vi "Main.vi"(11 "ROS_Master in":refnum<class "ROS_Master.lvclass">) -> ()   [LabVIEW 2013, in "ROS_Master.lvclass"]
uses:
  <userlib>/ROSforLV/ROS/Code/SubVIs/ROS_Master/ROS_Master.lvclass
  <userlib>/ROSforLV/ROS/Code/SubVIs/ROS_Master/ROS_Master.lvclass/ROS_Master.ctl
  <userlib>/ROSforLV/ROS/Code/_ROSDefinition.vi
panel:
  in  "stop":bool
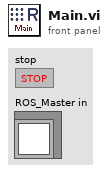
[diagram p1: front panel]
types:
  T1 = cluster{"Caller ID":string, "IP":string, "Msg Type":string, "Direction":enum16{"Publisher", "Subscriber"}, "Topic":string}
  T2 = cluster{"value":string, "value":string, "value":string}
  T3 = cluster{"Service":string, "Service IP":string, "Caller IP":string, "Caller ID":string}[]
  T4 = cluster{"Service":string, "Service IP":string, "Caller IP":string, "Caller ID":string}
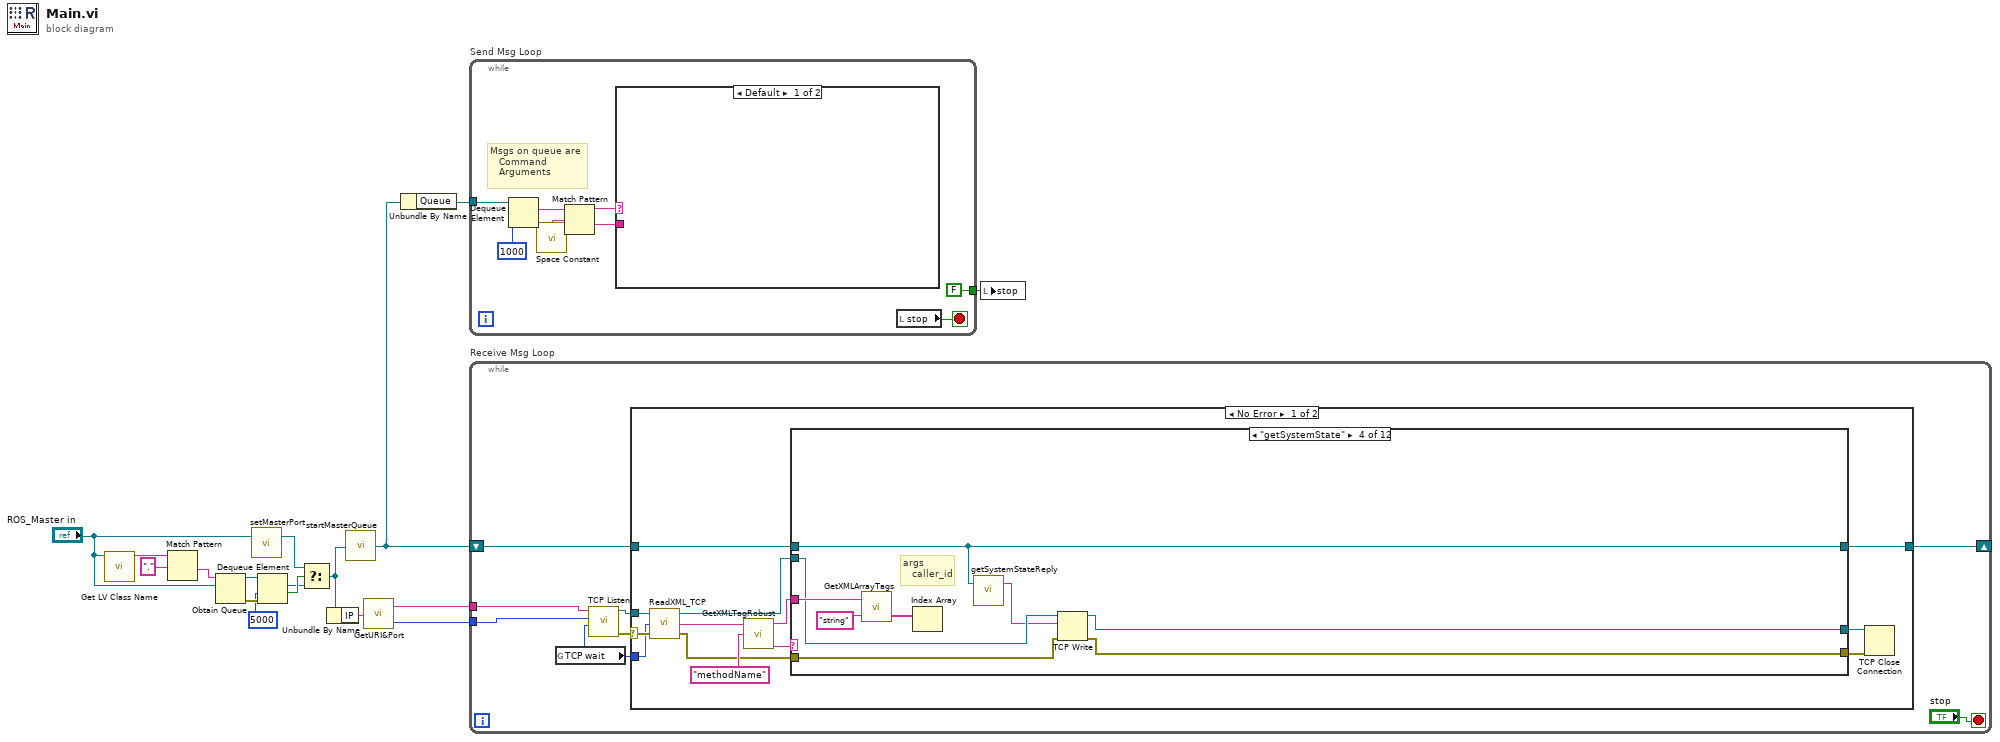
[diagram p0: block diagram]
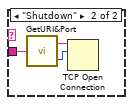
[diagram p2: hidden frame]
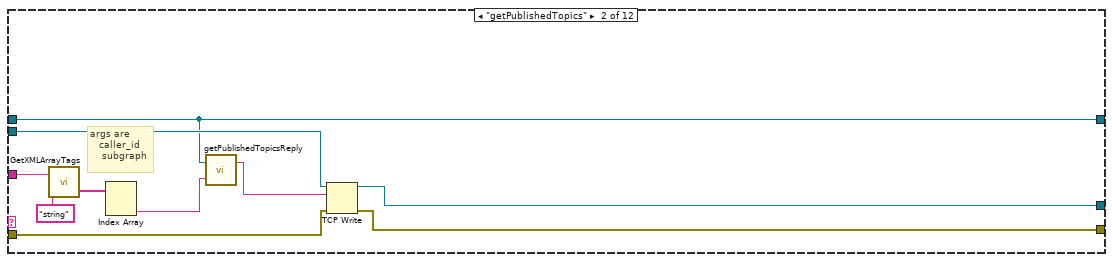
[diagram p4: hidden frame]
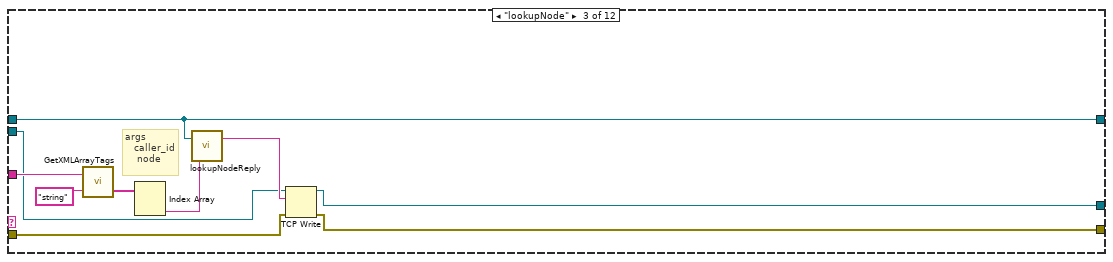
[diagram p5: hidden frame]
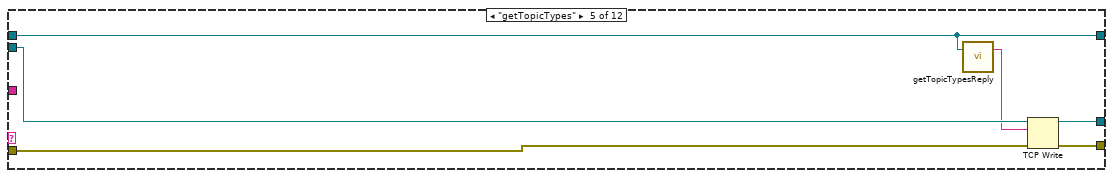
[diagram p6: hidden frame]
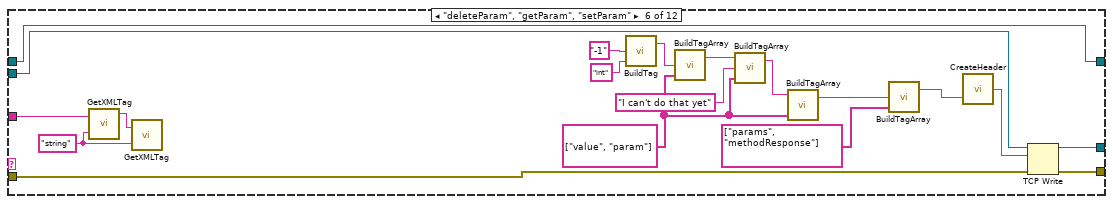
[diagram p7: hidden frame]
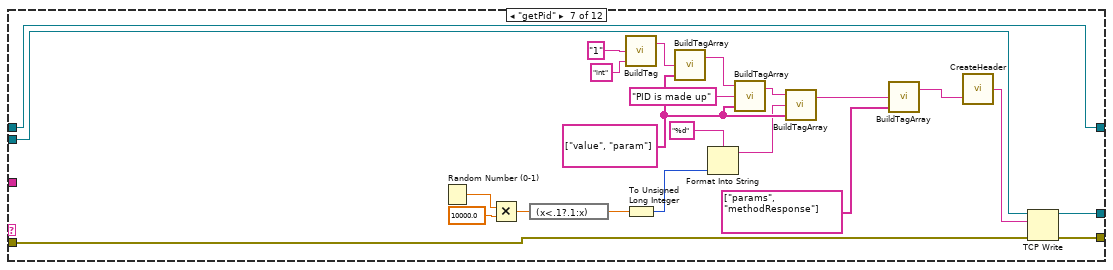
[diagram p8: hidden frame]
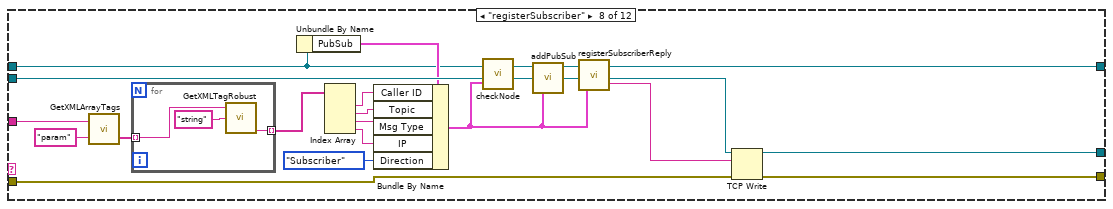
[diagram p9: hidden frame]
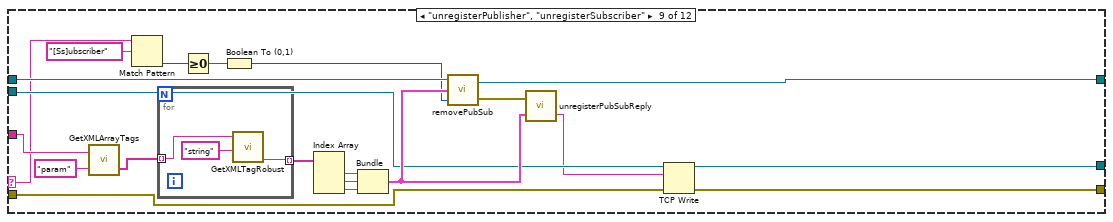
[diagram p10: hidden frame]
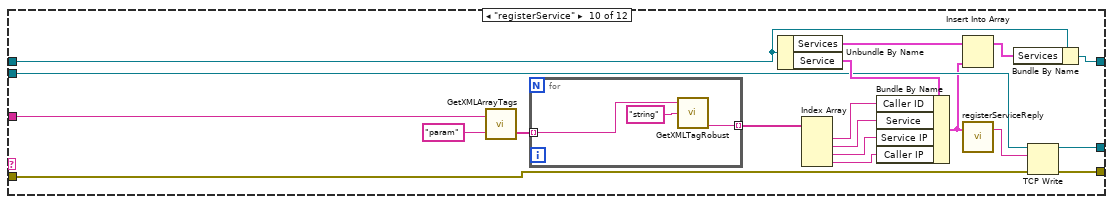
[diagram p11: hidden frame]
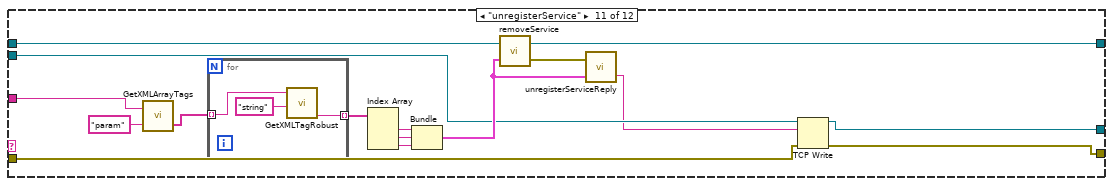
[diagram p12: hidden frame]
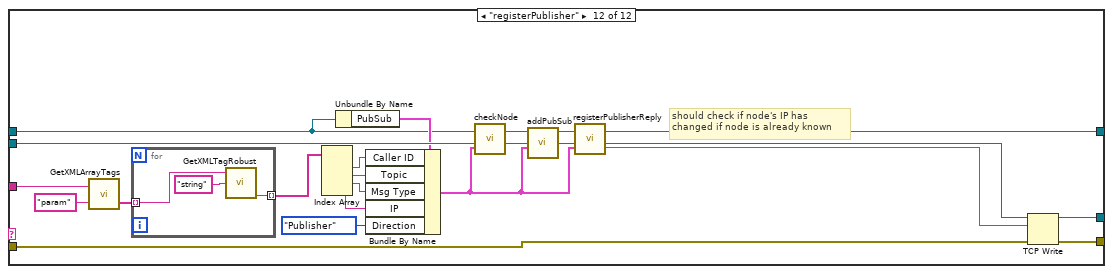
[diagram p13: hidden frame]
diagram:
  n1 = call <vilib>:"Get LV Class Name.vi"("object"="ROS_Master in") -> ("class name"=w14:string)  [unwired: 9 in, 1 out]
  n2 = Match Pattern(string=w14, regular expression=".") -> (after substring=w12:string)  [unwired: 1 in, 3 out]
  n3 = Obtain Queue(name (unnamed)=w12, element data type="ROS_Master in") -> (queue out=w10:refnum<queue>, error out=w11:errorcluster)  [unwired: 3 in, 1 out]
  n4 = call <userlib>:"setMasterPort.vi"("ROS_Master.lvclass in"="ROS_Master in") -> ("ROS_Master.lvclass out"=w6:refnum<class "ROS_Master.lvclass">)  [unwired: 2 in]
  n5 = Dequeue Element(queue=w10, timeout in ms (-1)=5000, error in (no error)=w11) -> (element=w5:refnum<class "ROS_Master.lvclass">, timed out?=w9:bool)  [unwired: 2 out]
  n6 = Select(t=w6, s=w9, f=w5) -> (s? t:f=w4:refnum<class "ROS_Master.lvclass">)
  n7 = Unbundle By Name(w4) -> ("IP"=w17:string)
  n8 = call <userlib>:"startMasterQueue.vi"("ROS_Master in"=w4) -> ("ROS_Master out"=w2:refnum<class "ROS_Master.lvclass">)
  n9 = call <userlib>:"GetURI&Port.vi"("URI in"=w17) -> ("Port"=w15:u16, "URI"=w16:string)
  n10 = Unbundle By Name(w2) -> ("Queue"=w1:refnum<queue>)
  n11 = while "Send Msg Loop" {
    tunnel: [FALSE ("stop")] -> w3
    tunnel: w1 -> [w23]
    stop <- w25 stop-if-true
    # "Msgs on queue are\n   Command\n   Arguments"
    n12 = Dequeue Element(queue=w23, timeout in ms (-1)=1000) -> (element=w21:string)  [unwired: 1 in, 3 out]
    n13 = call <vilib>:"Space Constant.vi"() -> ("String"=w20:string)
    n14 = Match Pattern(string=w21, regular expression=w20) -> (before substring=w19:string, after substring=w18:string)  [unwired: 1 in, 2 out]
    n15 = case shown="Default" w19 {
      tunnel: w18 -> [_ w28]
      frame Default {
      }
      frame "Shutdown" {
        n16 = call <userlib>:"GetURI&Port.vi"("URI in"=w28) -> ("Port"=w26:u16, "URI"=w27:string)
        n17 = TCP Open Connection(address=w27, remote port or service name=w26) -> ()  [unwired: 3 in, 2 out]
      }
    }
    n18 = local read "stop"() -> (w25:bool)
  }
  n19 = while "Receive Msg Loop" {
    shift-right: [w30] -> _
    shift-left: w2 -> [w31]
    tunnel: w16 -> [w34]
    tunnel: w15 -> [w33]
    stop <- "stop" stop-if-true
    n20 = global read "_ROSDefinition.vi" "TCP wait"() -> (w29:i32)
    n21 = call <vilib>:"TCP Listen.vi"("timeout ms (wait forever: -1)"=w29, "port"=w33, "service name"=w34) -> ("error out"=w35:errorcluster, "connection ID"=w32:refnum<k5>)  [unwired: 4 in, 3 out]
    n22 = case shown="No Error" w35 {
      selector: w35 -> [w48 _]
      tunnel: w32 -> [w49 _]
      tunnel: w31 -> [w43 w239]
      tunnel: [w42 w239] -> w30
      tunnel: w29 -> [w41 _]
      frame No Error {
        n23 = call <userlib>:"ReadXML_TCP.vi"("error in"=w48, "timeout ms (3000)"=w41, "connection ID in"=w49) -> ("error out"=w37:errorcluster, "data out"=w47:string, "connection ID out"=w40:refnum<k5>)
        n24 = call <userlib>:"GetXMLTagRobust.vi"("Tag"="methodName", "String"=w47) -> ("value"=w45:string, "String w/o Tag"=w44:string)  [unwired: 1 in, 2 out]
        n25 = case shown="\"getSystemState\"" w45 {
          selector: w45 -> [_ _ _ _ _ _ _ _ w156 _ _ _]
          tunnel: w44 -> [_ w62 w72 w81 _ w105 _ w148 w172 w194 w209 w235]
          tunnel: w43 -> [w52 w53 w63 w74 w82 w106 w129 w131 w165 w190 w206 w219]
          tunnel: [w52 w53 w63 w74 w82 w106 w129 w139 w164 w184 w198 w226] -> w42
          tunnel: w40 -> [w51 w58 w67 w78 w85 w92 w116 w144 w160 w181 w203 w231]
          tunnel: [w51 w55 w64 w75 w87 w90 w115 w143 w158 w179 w200 w229] -> w39
          tunnel: [w50 w54 w65 w76 w86 w89 w114 w141 w157 w178 w199 w228] -> w38
          tunnel: w37 -> [w50 w56 w66 w77 w84 w91 w113 w142 w161 w180 w202 w230]
          frame Default {
          }
          frame "getPublishedTopics" {
            # "args are\n   caller_id\n    subgraph"
            n26 = call <userlib>:"GetXMLArrayTags.vi"("ArrayTag"="string", "String"=w62) -> ("Array"=w60:string[])  [unwired: 1 out]
            n27 = Index Array(array=w60) -> (element #2=w59:string)  [unwired: 2 in, 1 out]
            n28 = call <userlib>:"getPublishedTopicsReply.vi"("Subgraph"=w59, "ROS_Master"=w53) -> ("XML"=w57:string)  [unwired: 1 in]
            n29 = TCP Write(connection ID=w58, data in=w57, error in (no error)=w56) -> (connection ID out=w55:refnum<k5>, error out=w54:errorcluster)  [unwired: 1 in, 1 out]
          }
          frame "lookupNode" {
            # "args\n   caller_id\n    node"
            n30 = call <userlib>:"GetXMLArrayTags.vi"("ArrayTag"="string", "String"=w72) -> ("Array"=w70:string[])  [unwired: 1 out]
            n31 = Index Array(array=w70) -> (element #2=w69:string)  [unwired: 2 in, 1 out]
            n32 = call <userlib>:"lookupNodeReply.vi"("node"=w69, "Master"=w63) -> ("XML"=w68:string)  [unwired: 1 in]
            n33 = TCP Write(connection ID=w67, data in=w68, error in (no error)=w66) -> (connection ID out=w64:refnum<k5>, error out=w65:errorcluster)  [unwired: 1 in, 1 out]
          }
          frame "getSystemState" {
            # "args\n   caller_id"
            n34 = call <userlib>:"GetXMLArrayTags.vi"("ArrayTag"="string", "String"=w81) -> ("Array"=w79:string[])  [unwired: 1 out]
            n35 = Index Array(array=w79) -> ()  [unwired: 1 in, 1 out]
            n36 = call <userlib>:"getSystemStateReply.vi"("ROS_Master in"=w74) -> ("XML"=w73:string)  [unwired: 2 in]
            n37 = TCP Write(connection ID=w78, data in=w73, error in (no error)=w77) -> (connection ID out=w75:refnum<k5>, error out=w76:errorcluster)  [unwired: 1 in, 1 out]
          }
          frame "getTopicTypes" {
            n38 = call <userlib>:"getTopicTypesReply.vi"("ROS_Master.lvclass in"=w82) -> ("Topics XML"=w83:string)  [unwired: 2 in]
            n39 = TCP Write(connection ID=w85, data in=w83, error in (no error)=w84) -> (connection ID out=w87:refnum<k5>, error out=w86:errorcluster)  [unwired: 1 in, 1 out]
          }
          frame "deleteParam", "getParam", "setParam" {
            w102 = string[] ["value", "param"] ("tags")
            w103 = "string" ("Tag")
            n40 = call <userlib>:"GetXMLTag.vi"("Tag"=w103, "String"=w105) -> ("String w/o Tag"=w104:string)  [unwired: 2 out]
            n41 = call <userlib>:"GetXMLTag.vi"("Tag"=w103, "String"=w104) -> ()  [unwired: 3 out]
            n42 = call <userlib>:"BuildTag.vi"("tag"="int", "value"="-1") -> ("string out"=w96:string)  [unwired: 2 in]
            n43 = call <userlib>:"BuildTagArray.vi"("tags"=w102, "value"=w96) -> ("string out"=w101:string)  [unwired: 2 in]
            n44 = call <userlib>:"BuildTagArray.vi"("tags"=w102, "value"="I can't do that yet", "string in"=w101) -> ("string out"=w100:string)  [unwired: 1 in]
            n45 = call <userlib>:"BuildTagArray.vi"("tags"=w102, "string in"=w100) -> ("string out"=w94:string)  [unwired: 2 in]
            n46 = call <userlib>:"BuildTagArray.vi"("tags"=string[] ["params", "methodResponse"], "value"=w94) -> ("string out"=w93:string)  [unwired: 2 in]
            n47 = call <userlib>:"CreateHeader.vi"("Content"=w93) -> ("XML"=w88:string)  [unwired: 1 in]
            n48 = TCP Write(connection ID=w92, data in=w88, error in (no error)=w91) -> (connection ID out=w90:refnum<k5>, error out=w89:errorcluster)  [unwired: 1 in, 1 out]
          }
          frame "getPid" {
            w128 = string[] ["value", "param"] ("tags")
            n49 = Random Number (0-1)() -> (number: 0 to 1=w125:dbl)
            n50 = Multiply(x=w125, y=10000.0) -> (x*y=w112:dbl)
            n51 = expression code="(x<.1?.1:x)"(w112) -> (w111:dbl)
            n52 = call <userlib>:"BuildTag.vi"("tag"="int", "value"="1") -> ("string out"=w107:string)  [unwired: 2 in]
            n53 = To Unsigned Long Integer(number=w111) -> (unsigned 32bit integer=w123:u32)
            n54 = call <userlib>:"BuildTagArray.vi"("tags"=w128, "value"=w107) -> ("string out"=w127:string)  [unwired: 2 in]
            n55 = Format Into String(format string="%d", w123) -> (resulting string=w121:string)  [unwired: 2 in, 1 out]
            n56 = call <userlib>:"BuildTagArray.vi"("tags"=w128, "value"="PID is made up", "string in"=w127) -> ("string out"=w126:string)  [unwired: 1 in]
            n57 = call <userlib>:"BuildTagArray.vi"("tags"=w128, "value"=w121, "string in"=w126) -> ("string out"=w120:string)  [unwired: 1 in]
            n58 = call <userlib>:"BuildTagArray.vi"("tags"=string[] ["params", "methodResponse"], "value"=w120) -> ("string out"=w118:string)  [unwired: 2 in]
            n59 = call <userlib>:"CreateHeader.vi"("Content"=w118) -> ("XML"=w117:string)  [unwired: 1 in]
            n60 = TCP Write(connection ID=w116, data in=w117, error in (no error)=w113) -> (connection ID out=w115:refnum<k5>, error out=w114:errorcluster)  [unwired: 1 in, 1 out]
          }
          frame "registerSubscriber" {
            n61 = call <userlib>:"GetXMLArrayTags.vi"("ArrayTag"="param", "String"=w148) -> ("Array"=w146:string[])  [unwired: 1 out]
            n62 = for {
              tunnel: w146 -> [w151] mode=indexing
              tunnel: [w149] -> w145 mode=indexing
              n63 = call <userlib>:"GetXMLTagRobust.vi"("Tag"="string", "String"=w151) -> ("value"=w149:string)  [unwired: 1 in, 3 out]
            }
            n64 = Unbundle By Name(w131) -> ("PubSub"=w134:T1)
            n65 = Index Array(array=w145) -> (element #1=w138:string, element #2=w137:string, element #3=w136:string, element #4=w135:string)  [unwired: 4 in]
            n66 = Bundle By Name(cluster=w134, "Caller ID"=w138, "Topic"=w137, "Msg Type"=w136, "IP"=w135, "Direction"=enum16{"Publisher", "Subscriber"}."Subscriber") -> (w132:T1)
            n67 = call <userlib>:"checkNode.vi"("PubSub"=w132, "ROS_Master"=w131) -> ("ROS_Master out"=w130:refnum<class "ROS_Master.lvclass">)  [unwired: 1 in]
            n68 = call <userlib>:"addPubSub.vi"("PubSub"=w132, "ROS_Master in"=w130) -> ("ROS_Master out"=w139:refnum<class "ROS_Master.lvclass">)  [unwired: 9 in]
            n69 = call <userlib>:"registerSubscriberReply.vi"("Subscriber"=w132, "ROS_Master.lvclass in"=w139) -> ("XML"=w140:string)  [unwired: 1 in]
            n70 = TCP Write(connection ID=w144, data in=w140, error in (no error)=w142) -> (connection ID out=w143:refnum<k5>, error out=w141:errorcluster)  [unwired: 1 in, 1 out]
          }
          frame "unregisterPublisher", "unregisterSubscriber" {
            n71 = call <userlib>:"GetXMLArrayTags.vi"("ArrayTag"="param", "String"=w172) -> ("Array"=w170:string[])  [unwired: 1 out]
            n72 = Match Pattern(string=w156, regular expression="[Ss]ubscriber") -> (offset past match=w154:i32)  [unwired: 1 in, 3 out]
            n73 = for {
              tunnel: w170 -> [w175] mode=indexing
              tunnel: [w173] -> w169 mode=indexing
              n74 = call <userlib>:"GetXMLTagRobust.vi"("Tag"="string", "String"=w175) -> ("value"=w173:string)  [unwired: 1 in, 3 out]
            }
            n75 = Greater Or Equal To 0?(x=w154) -> (x >= 0?=w153:bool)
            n76 = Boolean To (0,1)(Boolean=w153) -> (0, 1=w152:i16)
            n77 = Index Array(array=w169) -> (element #1=w168:string, element #2=w167:string, element #3=w166:string)  [unwired: 3 in]
            n78 = Bundle("value"=w168, "value"=w167, "value"=w166) -> (w163:T2)  [unwired: 1 in]
            n79 = call <userlib>:"removePubSub.vi"("Direction"=w152, "PubSub"=w163, "ROS_Master in"=w165) -> ("error out"=w162:errorcluster, "ROS_Master out"=w164:refnum<class "ROS_Master.lvclass">)
            n80 = call <userlib>:"unregisterPubSubReply.vi"("PubSub"=w163, "error in"=w162) -> ("XML"=w159:string)  [unwired: 1 in]
            n81 = TCP Write(connection ID=w160, data in=w159, error in (no error)=w161) -> (connection ID out=w158:refnum<k5>, error out=w157:errorcluster)  [unwired: 1 in, 1 out]
          }
          frame "registerService" {
            n82 = call <userlib>:"GetXMLArrayTags.vi"("ArrayTag"="param", "String"=w194) -> ("Array"=w192:string[])  [unwired: 1 out]
            n83 = for {
              tunnel: w192 -> [w197] mode=indexing
              tunnel: [w195] -> w191 mode=indexing
              n84 = call <userlib>:"GetXMLTagRobust.vi"("Tag"="string", "String"=w197) -> ("value"=w195:string)  [unwired: 1 in, 3 out]
            }
            n85 = Unbundle By Name(w190) -> ("Services"=w185:T3, "Service"=w189:T4)
            n86 = Index Array(array=w191) -> (element #1=w188:string, element #2=w187:string, element #3=w186:string, element #4=w183:string)  [unwired: 4 in]
            n87 = Bundle By Name(cluster=w189, "Caller ID"=w188, "Service"=w187, "Service IP"=w186, "Caller IP"=w183) -> (w177:T4)
            n88 = Insert Into Array(array=w185, new element=w177) -> (w182:T3)  [unwired: 1 in]
            n89 = call <userlib>:"registerServiceReply.vi"("Service"=w177) -> ("XML"=w176:string)  [unwired: 2 in]
            n90 = Bundle By Name(cluster=w190, "Services"=w182) -> (w184:refnum<class "ROS_Master.lvclass">)
            n91 = TCP Write(connection ID=w181, data in=w176, error in (no error)=w180) -> (connection ID out=w179:refnum<k5>, error out=w178:errorcluster)  [unwired: 1 in, 1 out]
          }
          frame "unregisterService" {
            n92 = call <userlib>:"GetXMLArrayTags.vi"("ArrayTag"="param", "String"=w209) -> ("Array"=w208:string[])  [unwired: 1 out]
            n93 = for {
              tunnel: w208 -> [w215] mode=indexing
              tunnel: [w214] -> w207 mode=indexing
              n94 = call <userlib>:"GetXMLTagRobust.vi"("Tag"="string", "String"=w215) -> ("value"=w214:string)  [unwired: 1 in, 3 out]
            }
            n95 = Index Array(array=w207) -> (element #1=w212:string, element #2=w211:string, element #3=w210:string)  [unwired: 3 in]
            n96 = Bundle("value"=w212, "value"=w211, "value"=w210) -> (w204:T2)  [unwired: 1 in]
            n97 = call <userlib>:"removeService.vi"("Service"=w204, "ROS_Master in"=w206) -> ("error out"=w205:errorcluster, "ROS_Master out"=w198:refnum<class "ROS_Master.lvclass">)
            n98 = call <userlib>:"unregisterServiceReply.vi"("Service"=w204, "error in"=w205) -> ("XML"=w201:string)  [unwired: 1 in]
            n99 = TCP Write(connection ID=w203, data in=w201, error in (no error)=w202) -> (connection ID out=w200:refnum<k5>, error out=w199:errorcluster)  [unwired: 1 in, 1 out]
          }
          frame "registerPublisher" {
            # "should check if node's IP has \nchanged if node is already known"
            n100 = call <userlib>:"GetXMLArrayTags.vi"("ArrayTag"="param", "String"=w235) -> ("Array"=w233:string[])  [unwired: 1 out]
            n101 = for {
              tunnel: w233 -> [w238] mode=indexing
              tunnel: [w236] -> w232 mode=indexing
              n102 = call <userlib>:"GetXMLTagRobust.vi"("Tag"="string", "String"=w238) -> ("value"=w236:string)  [unwired: 1 in, 3 out]
            }
            n103 = Index Array(array=w232) -> (element #1=w225:string, element #2=w224:string, element #3=w223:string, element #4=w222:string)  [unwired: 4 in]
            n104 = Unbundle By Name(w219) -> ("PubSub"=w221:T1)
            n105 = Bundle By Name(cluster=w221, "Caller ID"=w225, "Topic"=w224, "Msg Type"=w223, "IP"=w222, "Direction"=enum16{"Publisher", "Subscriber"}."Publisher") -> (w218:T1)
            n106 = call <userlib>:"checkNode.vi"("PubSub"=w218, "ROS_Master"=w219) -> ("ROS_Master out"=w217:refnum<class "ROS_Master.lvclass">)  [unwired: 1 in]
            n107 = call <userlib>:"addPubSub.vi"("PubSub"=w218, "ROS_Master in"=w217) -> ("ROS_Master out"=w226:refnum<class "ROS_Master.lvclass">)  [unwired: 9 in]
            n108 = call <userlib>:"registerPublisherReply.vi"("Publisher"=w218, "ROS_Master.lvclass in"=w226) -> ("XML"=w227:string)  [unwired: 1 in]
            n109 = TCP Write(connection ID=w231, data in=w227, error in (no error)=w230) -> (connection ID out=w229:refnum<k5>, error out=w228:errorcluster)  [unwired: 1 in, 1 out]
          }
        }
        n110 = TCP Close Connection(connection ID=w39, error in (no error)=w38) -> ()  [unwired: 1 in, 2 out]
      }
      frame Error {
      }
    }
  }
  n111 = local write "stop"(w3) -> ()
